vi "Load DAC Configuration.vi"(8 "error in":errorcluster, 10 "Config File refnum in":T1, 11 "DAC Traverse in":refnum<class "DAC Traverse.lvclass">) -> (0 "error out":errorcluster, 2 "Config File refnum out":T1, 3 "DAC Traverse out":refnum<class "DAC Traverse.lvclass">)   [LabVIEW 2019, in "DAC.lvlib" / "DAC Traverse.lvclass"]
uses:
  DAC Traverse.lvclass
  <vilib>/Utility/config.llb/NI_LVConfig.lvlib
  <vilib>/Utility/config.llb/Read Key (String).vi
  DAC.lvclass
  C:/Users/wg/Documents/LV_Projects/test-stand/App/DAC/DAC.lvclass
  <vilib>/Utility/config.llb/Config Data RefNum.ctl
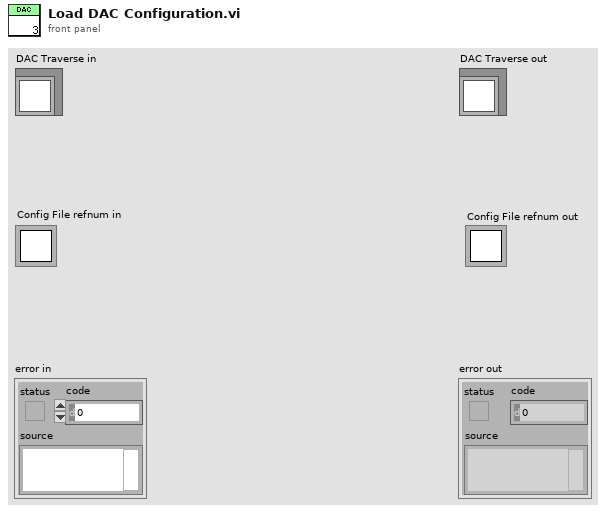
[diagram p1: front panel]
types:
  T1 = typedef "NI_LVConfig.lvlib/Config Data RefNum.ctl" = refnum<k1>
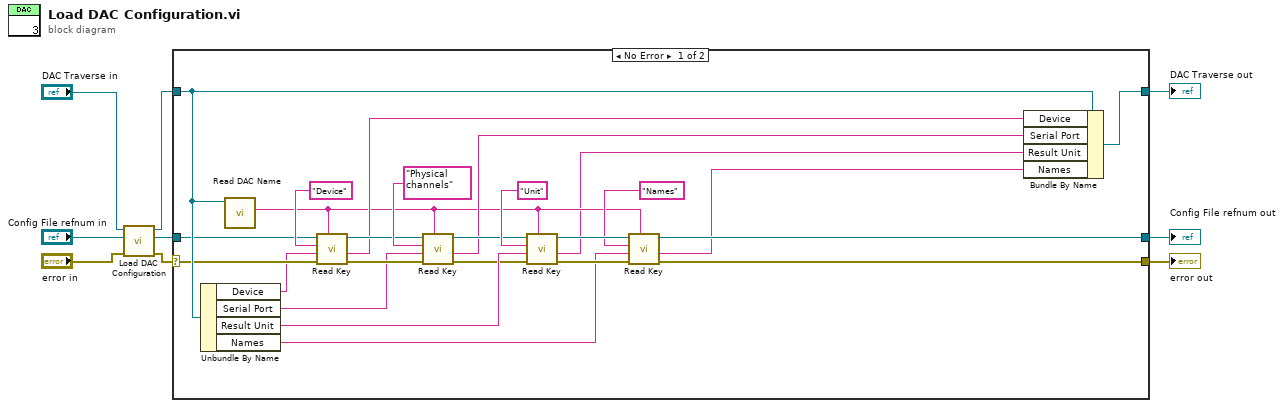
[diagram p0: block diagram]
diagram:
  n1 = call-parent "Load DAC Configuration.vi"("error in"="error in", "Config File refnum in"="Config File refnum in", "DAC in"="DAC Traverse in") -> ("error out"=w4:errorcluster, "Config File refnum out"=w5:T1, "DAC out"=w6:refnum<class "DAC Traverse.lvclass">)  [unwired: 6 in]
  n2 = case shown="No Error" w4 {
    selector: w4 -> [w22 w35]
    tunnel: [w30 w37] -> w3
    tunnel: w6 -> [w29 w37]
    tunnel: w5 -> [w23 w36]
    tunnel: [w12 w36] -> w2
    tunnel: [w13 w35] -> w1
    frame No Error {
      n3 = Unbundle By Name(w29) -> ("Device"=w18:string, "Serial Port"=w17:string, "Result Unit"=w28:string, "Names"=w27:string)
      n4 = call "Read DAC Name.vi"("DAC in"=w29) -> ("DAC Name"=w14:string)  [unwired: 8 in, 2 out]
      n5 = call-poly <vilib>:"Read Key.vi"("section"=w14, "error in (no error)"=w22, "default value"=w18, "key"="Device", "refnum"=w23) -> ("error out"=w21:errorcluster, "value"=w16:string, "refnum out"=w24:T1)  [unwired: 3 in, 1 out]
      n6 = call-poly <vilib>:"Read Key.vi"("section"=w14, "error in (no error)"=w21, "default value"=w17, "key"="Physical channels", "refnum"=w24) -> ("error out"=w19:errorcluster, "value"=w15:string, "refnum out"=w20:T1)  [unwired: 3 in, 1 out]
      n7 = call-poly <vilib>:"Read Key.vi"("section"=w14, "error in (no error)"=w19, "default value"=w28, "key"="Unit", "refnum"=w20) -> ("error out"=w33:errorcluster, "value"=w11:string, "refnum out"=w34:T1)  [unwired: 3 in, 1 out]
      n8 = call-poly <vilib>:"Read Key.vi"("section"=w14, "error in (no error)"=w33, "default value"=w27, "key"="Names", "refnum"=w34) -> ("error out"=w13:errorcluster, "value"=w10:string, "refnum out"=w12:T1)  [unwired: 3 in, 1 out]
      n9 = Bundle By Name(cluster=w29, "Device"=w16, "Serial Port"=w15, "Result Unit"=w11, "Names"=w10) -> (w30:refnum<class "DAC Traverse.lvclass">)
    }
    frame Error {
    }
  }
  "error out" <- w1
  "DAC Traverse out" <- w3
  "Config File refnum out" <- w2
